vi "Drive Mode Cleaned.vi"   [LabVIEW 2018]
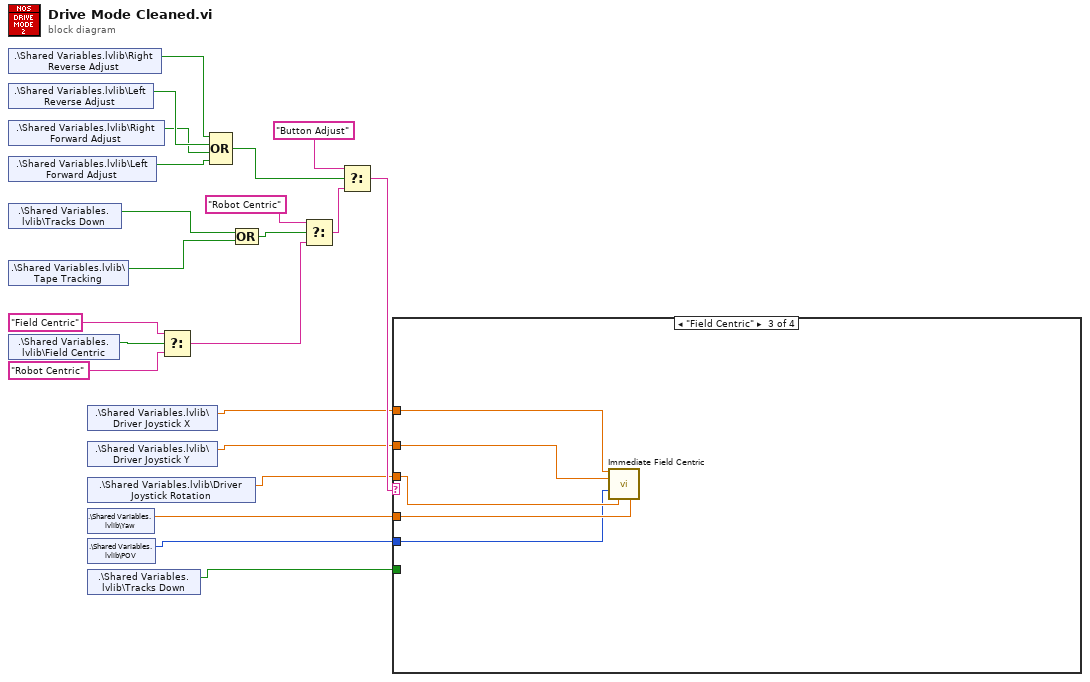
[diagram p0: block diagram]
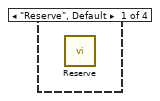
[diagram p2: hidden frame]
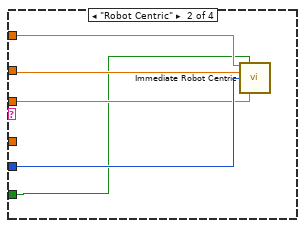
[diagram p3: hidden frame]
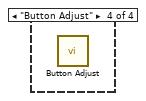
[diagram p4: hidden frame]
diagram:
  n1 = shared-variable ".\\Shared Variables.lvlib\\Right Reverse Adjust"() -> (w8:bool)  [unwired: 1 in, 1 out]
  n2 = shared-variable ".\\Shared Variables.lvlib\\Left Reverse Adjust"() -> (w7:bool)  [unwired: 1 in, 1 out]
  n3 = shared-variable ".\\Shared Variables.lvlib\\Right Forward Adjust"() -> (w6:bool)  [unwired: 1 in, 1 out]
  n4 = shared-variable ".\\Shared Variables.lvlib\\Left Forward Adjust"() -> (w5:bool)  [unwired: 1 in, 1 out]
  n5 = shared-variable ".\\Shared Variables.lvlib\\Tracks Down"() -> (w3:bool)  [unwired: 1 in, 1 out]
  n6 = shared-variable ".\\Shared Variables.lvlib\\Tape Tracking"() -> (w2:bool)  [unwired: 1 in, 1 out]
  n7 = shared-variable ".\\Shared Variables.lvlib\\Field Centric"() -> (w21:bool)  [unwired: 1 in, 1 out]
  n8 = shared-variable ".\\Shared Variables.lvlib\\Driver Joystick X"() -> (w17:dbl)  [unwired: 1 in, 1 out]
  n9 = shared-variable ".\\Shared Variables.lvlib\\Driver Joystick Y"() -> (w16:dbl)  [unwired: 1 in, 1 out]
  n10 = shared-variable ".\\Shared Variables.lvlib\\Driver Joystick Rotation"() -> (w15:dbl)  [unwired: 1 in, 1 out]
  n11 = shared-variable ".\\Shared Variables.lvlib\\Yaw"() -> (w14:dbl)  [unwired: 1 in, 1 out]
  n12 = shared-variable ".\\Shared Variables.lvlib\\POV"() -> (w13:i16)  [unwired: 1 in, 1 out]
  n13 = shared-variable ".\\Shared Variables.lvlib\\Tracks Down"() -> (w12:bool)  [unwired: 1 in, 1 out]
  n14 = Select(t="Field Centric", s=w21, f="Robot Centric") -> (s? t:f=w10:string)
  n15 = Compound Arithmetic op=OR(w8, w7, w6, w5) -> (w4:bool)
  n16 = Compound Arithmetic op=OR(w3, w2) -> (w1:bool)
  n17 = Select(t="Robot Centric", s=w1, f=w10) -> (s? t:f=w11:string)
  n18 = Select(t="Button Adjust", s=w4, f=w11) -> (s? t:f=w18:string)
  n19 = case shown="\"Field Centric\"" w18 {
    tunnel: w17 -> [_ w27 w32 _]
    tunnel: w16 -> [_ w26 w31 _]
    tunnel: w15 -> [_ w24 w29 _]
    tunnel: w14 -> [_ _ w30 _]
    tunnel: w13 -> [_ w25 w28 _]
    tunnel: w12 -> [_ w23 _ _]
    frame "Reserve", Default {
      n20 = call "Reserve.vi"() -> ()  [unwired: 11 in, 1 out]
    }
    frame "Robot Centric" {
      n21 = call "Immediate Robot Centric.vi"("X Setpoint"=w27, "Tracks"=w23, "Y Setpoint"=w26, "POV"=w25, "Z Setpoint"=w24) -> ()  [unwired: 10 in, 1 out]
    }
    frame "Field Centric" {
      n22 = call "Immediate Field Centric.vi"("X Setpoint"=w32, "Y Setpoint"=w31, "POV"=w28, "Z Setpoint"=w29, "Gyro"=w30) -> ()  [unwired: 10 in, 1 out]
    }
    frame "Button Adjust" {
      n23 = call "Button Adjust.vi"() -> ()  [unwired: 11 in, 1 out]
    }
  }
